vi "Scale Inches to Encoder Counts.vi"(11 "Target Height (in)":dbl) -> (3 "Encoder Counts":dbl)   [LabVIEW 2017]
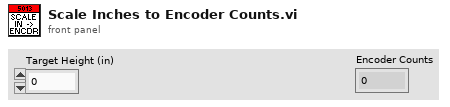
[diagram p1: front panel]
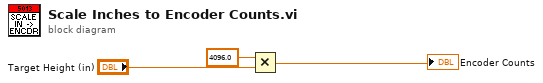
[diagram p0: block diagram]
diagram:
  n1 = Multiply(x=4096.0, y="Target Height (in)") -> (x*y=→"Encoder Counts":dbl)
